vi "YOLOv8_OpenVINO.vi"() -> ()   [LabVIEW 2018]
doc: "YOLOv8_OpenVINO: This example is an object detection example of YOLOv8 algorithm, which can perform object detection function on real-time images captured by cameras."
uses:
  vi.lib/VIRobotics/ModelZoo/Object_Detection/yolov8_openvino/InitialModel_yolov8_OpenVINO.vi
  vi.lib/VIRobotics/opencv_yiku/Cap/Cap.lvclass
  vi.lib/VIRobotics/ModelZoo/Object_Detection/yolov8_openvino/yolov8_openvino.lvclass
  vi.lib/VIRobotics/opencv_yiku/Mat/Mat_8U/Mat_8U.lvclass
panel:
  in  "device_name":string(combo)="CPU"
  in  "config":T1={"confThreshold"=0.3, "nms_threshold"=0.5, "fontScale"=0.5}
  out "每帧耗时(s)":dbl
  in  "class_names_file":path=path "C:/ProgramData/VIRobotics/ModelZoo/Object_Detection/coco.names"
  in  "model_file":path=path "C:/ProgramData/VIRobotics/ModelZoo/Object_Detection/yolov8/onnx_model/yolov8n.onnx"
  in  "stop":bool
  out "picture":picture
  # "Overview: Demonstrates how to use OpenVINO to load the the ONNX model of yolov8 for real-time object detection.\nRequirements: Windows.\nMake sure your computer has a camera。\nInstructions: \n1.Select the device_name to use.（If your computer has Intel GPU, you can select GPU in the \"type\" control before running the VI to achieve faster inference).\n2.Run the VI.\nIf you want to load the model you trained, follow the following steps:\n1.Select the device_name to use. \n2.Specify the model_file and class_names_file.\n3.Run the VI."
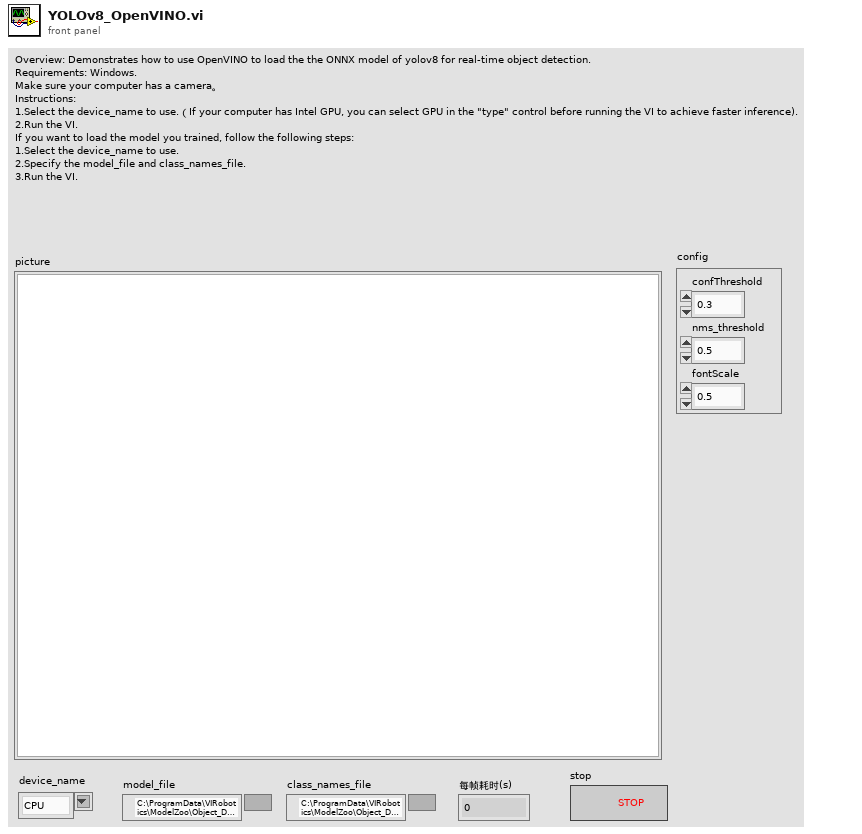
[diagram p1: front panel]
types:
  T1 = cluster{"confThreshold":sgl, "nms_threshold":sgl, "fontScale":dbl}
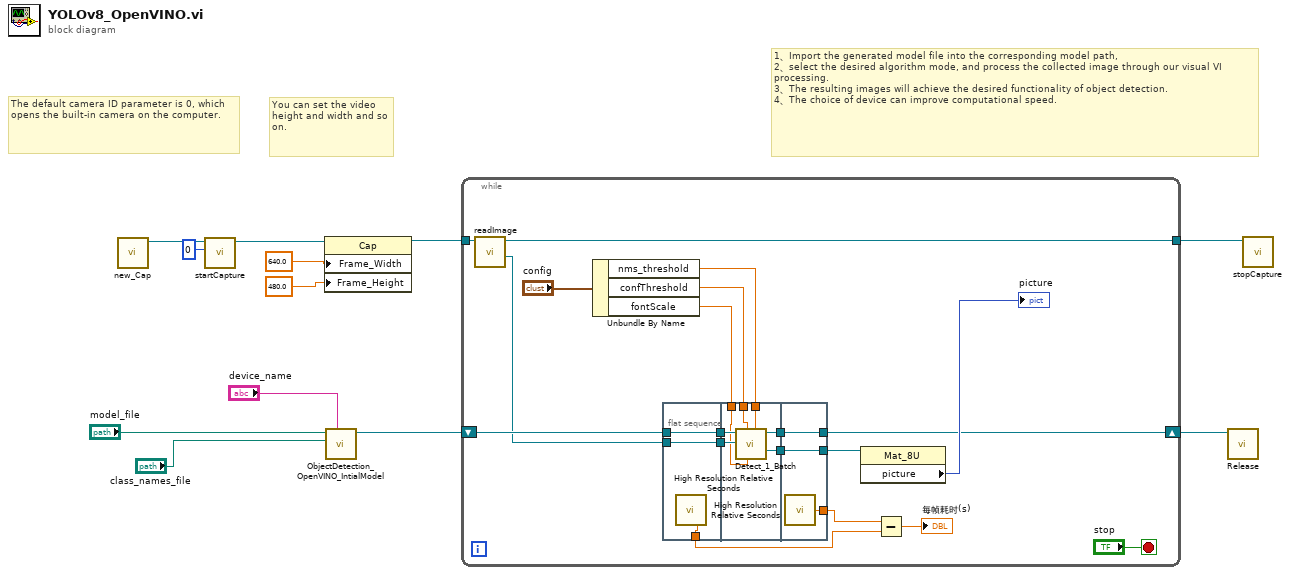
[diagram p0: block diagram]
diagram:
  # "1、Import the generated model file into the corresponding model path, \n2、select the desired algorithm mode, and process the collected image through our visual VI processing. \n3、The resulting images will achieve the desired functionality of object detection. \n4、The choice of device can improve computational speed."
  # "You can set the video height and width and so on."
  # "The default camera ID parameter is 0, which opens the built-in camera on the computer."
  n1 = call "new_Cap.vi"() -> ("Cap out"=w7:refnum<class "Cap.lvclass">)  [unwired: 10 in, 1 out]
  n2 = call "startCapture.vi"("cameraID"=0, "Cap in"=w7) -> ("Cap out"=w4:refnum<class "Cap.lvclass">)  [unwired: 8 in, 1 out]
  n3 = property class="Cap"(reference=w4, "Frame_Width"=640.0, "Frame_Height"=480.0) -> (reference out=w2:refnum<class "Cap.lvclass">)  [unwired: 1 in, 1 out]
  n4 = call-poly "ObjectDetection_OpenVINO_IntialModel.vi"("device_name"="device_name", "class_names_path"="class_names_file", "path"="model_file") -> ("yolov8_openvino out"=w10:refnum<class "yolov8_openvino.lvclass">)  [unwired: 7 in, 1 out]
  n5 = while {
    tunnel: w2 -> [w30]
    shift-right: [w26] -> w11
    shift-left: w10 -> [w31]
    tunnel: [w25] -> w12
    stop <- "stop" stop-if-true
    n6 = call "readImage.vi"("Cap in"=w30) -> ("Mat out"=w18:refnum<class "Mat_8U.lvclass">, "Cap out"=w25:refnum<class "Cap.lvclass">)  [unwired: 8 in, 1 out]
    n7 = Unbundle By Name("config") -> ("nms_threshold"=w15:sgl, "confThreshold"=w14:sgl, "fontScale"=w13:dbl)
    n8 = flat-sequence {
      tunnel: w31 -> [w34]
      tunnel: [w34] -> w24
      tunnel: [w33] -> w20
      tunnel: w18 -> [w32]
      tunnel: [w32] -> w17
      tunnel: w24 -> [w41]
      tunnel: [w40] -> w23
      tunnel: [w39] -> w22
      tunnel: w17 -> [w38]
      tunnel: w15 -> [w37]
      tunnel: w14 -> [w36]
      tunnel: w13 -> [w35]
      tunnel: [w43] -> w26
      tunnel: [w44] -> w29
      tunnel: w23 -> [w44]
      tunnel: w22 -> [w43]
      tunnel: [w42] -> w21
      frame #0 {
        n9 = call <vilib>:"High Resolution Relative Seconds.vi"() -> ("relative seconds"=w33:dbl)
      }
      frame #1 {
        n10 = call-dynamic "Detect_1_Batch.vi"("nms_threshold"=w37, "fontScale"=w35, "confThreshold"=w36, "image"=w38, "yolov8_openvino in"=w41) -> ("img out"=w40:refnum<class "Mat_8U.lvclass">, "yolov8_openvino out"=w39:refnum<class "yolov8_openvino.lvclass">)  [unwired: 3 in, 2 out]
      }
      frame #2 {
        n11 = call <vilib>:"High Resolution Relative Seconds.vi"() -> ("relative seconds"=w42:dbl)
      }
    }
    n12 = property class="Mat_8U"(reference=w29) -> ("picture"=→"picture":picture)  [unwired: 1 in, 2 out]
    n13 = Subtract(x=w21, y=w20) -> (x-y=→"每帧耗时(s)":dbl)
  }
  n14 = call-dynamic "Release.vi"("yolov8_openvino in"=w11) -> ()  [unwired: 9 in, 2 out]
  n15 = call "stopCapture.vi"("Cap in"=w12) -> ()  [unwired: 10 in, 1 out]
